vi "IsPDA.vi"   [LabVIEW 2015]
uses:
  ESLSCDLL.dll
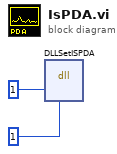
[diagram p0: block diagram]
diagram:
  n1 = dll-call lib="C:/ENTW/PCIE/64bit/lv64/lv15_act2018/board.vis/ESLSCDLL.dll" fn="DLLSetISPDA"("drv"=u32 1, "set"=u8 1) -> ()  [unwired: 6 in, 2 out]
